vi "例13.2 仿真信号的生成.vi"() -> ()   [LabVIEW 2017]
uses:
  <vilib>/measure/NI_MABase.lvlib
  <vilib>/measure/NI_MAPro.lvlib
panel:
  in  "相位":dbl
  in  "幅值":dbl
  in  "频率":dbl
  in  "停止":bool
  in  "formula":string="sin(w*t)*sin(2*pi(1)*t)" caption="公式"
  in  "噪声选择":enum16{"无", "均匀白噪声", "高斯噪声"}(ring)
  in  "波形选择":enum16{"正弦波", "三角波", "方波", "公式波"}(ring)
  in  "信噪比":dbl=1.0 format="%.2p"
  in  "square wave \nduty cycle (%)":dbl=50.0 caption="方波占空比(%)" format="%0.2f"
  in  "sampling info":cluster{"Fs":dbl, "#s":dbl}={"Fs"=1000.0, "#s"=1000.0} caption="采样信息" {"Fs" format="%.2p"}
  out "波形图":waveform(dbl)(graph)
  # "波 形 发 生 器"
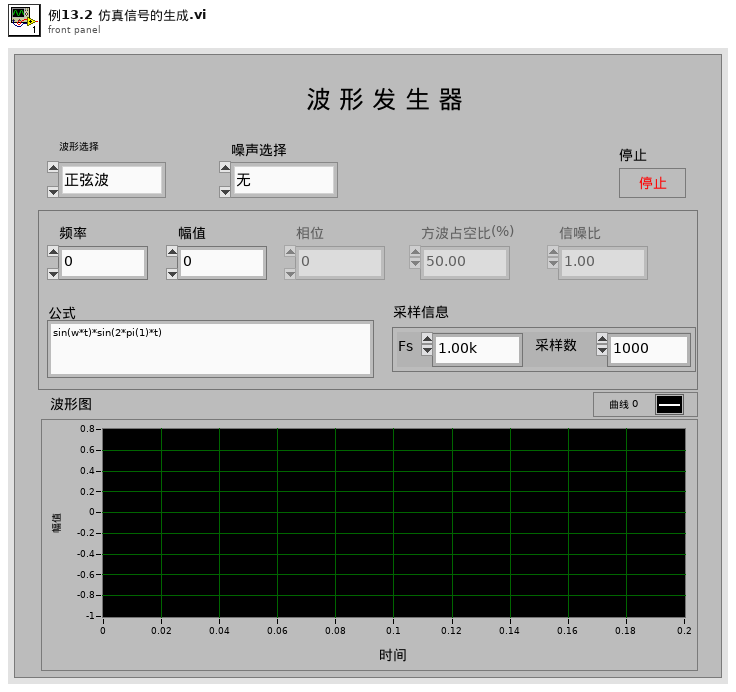
[diagram p1: front panel]
types:
  T1 = enum8{"Enabled", "Disabled", "Disabled and Grayed Out"}
  T2 = enum16{"Sine Wave", "Triangle Wave", "Square Wave", "Sawtooth Wave"}
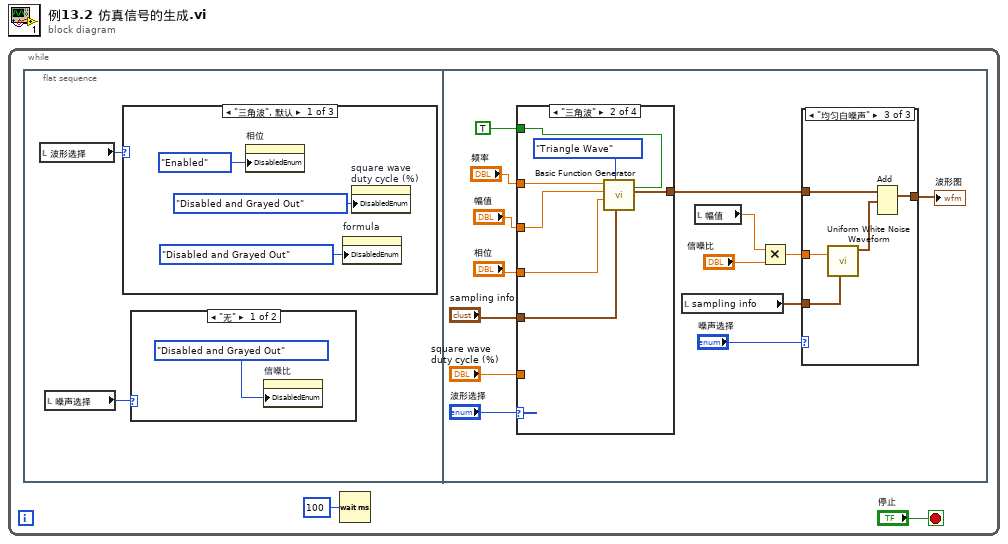
[diagram p0: block diagram]
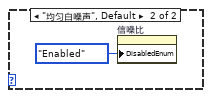
[diagram p2: hidden frame]
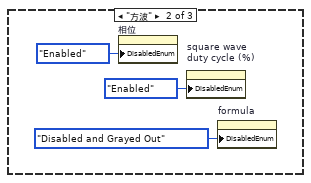
[diagram p3: hidden frame]
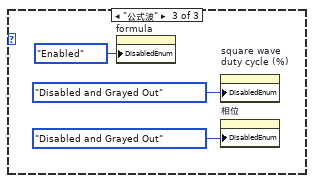
[diagram p4: hidden frame]
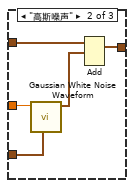
[diagram p6: hidden frame]
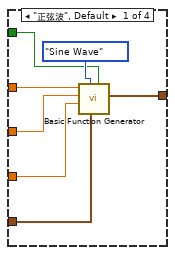
[diagram p7: hidden frame]
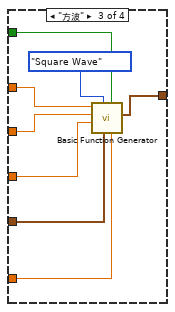
[diagram p8: hidden frame]
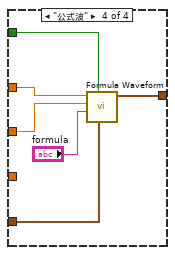
[diagram p9: hidden frame]
diagram:
  n1 = while {
    stop <- "停止" stop-if-true
    n2 = flat-sequence {
      frame #0 {
        n3 = local read "波形选择"() -> (w4:enum16{"正弦波", "三角波", "方波", "公式波"})
        n4 = local read "噪声选择"() -> (w3:enum16{"无", "均匀白噪声", "高斯噪声"})
        n5 = case shown="\"三角波\", 默认" w4 {
          frame "三角波", Default {
            n6 = property on="相位" class="DigNum (严格)"("DisabledEnum"=T1."Enabled" ("禁用")) -> ()  [unwired: 2 in, 2 out]
            n7 = property on="formula" class="Str"("DisabledEnum"=T1."Disabled and Grayed Out" ("禁用")) -> ()  [unwired: 2 in, 2 out]
            n8 = property on="square wave \nduty cycle (%)" class="DigNum (严格)"("DisabledEnum"=T1."Disabled and Grayed Out" ("禁用")) -> ()  [unwired: 2 in, 2 out]
          }
          frame "方波" {
            n9 = property on="相位" class="DigNum (严格)"("DisabledEnum"=T1."Enabled" ("禁用")) -> ()  [unwired: 2 in, 2 out]
            n10 = property on="square wave \nduty cycle (%)" class="DigNum (严格)"("DisabledEnum"=T1."Enabled" ("禁用")) -> ()  [unwired: 2 in, 2 out]
            n11 = property on="formula" class="Str"("DisabledEnum"=T1."Disabled and Grayed Out" ("禁用")) -> ()  [unwired: 2 in, 2 out]
          }
          frame "公式波" {
            n12 = property on="formula" class="Str"("DisabledEnum"=T1."Enabled" ("禁用")) -> ()  [unwired: 2 in, 2 out]
            n13 = property on="square wave \nduty cycle (%)" class="DigNum (严格)"("DisabledEnum"=T1."Disabled and Grayed Out" ("禁用")) -> ()  [unwired: 2 in, 2 out]
            n14 = property on="相位" class="DigNum (严格)"("DisabledEnum"=T1."Disabled and Grayed Out" ("禁用")) -> ()  [unwired: 2 in, 2 out]
          }
        }
        n15 = case shown="\"无\"" w3 {
          frame "无" {
            n16 = property on="信噪比" class="DigNum (严格)"("DisabledEnum"=T1."Disabled and Grayed Out" ("禁用")) -> ()  [unwired: 2 in, 2 out]
          }
          frame "均匀白噪声", Default {
            n17 = property on="信噪比" class="DigNum (严格)"("DisabledEnum"=T1."Enabled" ("禁用")) -> ()  [unwired: 2 in, 2 out]
          }
        }
      }
      frame #1 {
        n18 = case shown="\"三角波\"" "波形选择" {
          tunnel: [w43 w54 w56 w65] -> w27
          tunnel: "频率" -> [w46 w52 w61 w68]
          tunnel: "幅值" -> [w45 w51 w60 w67]
          tunnel: "相位" -> [w42 w50 w59 _]
          tunnel: "sampling info" -> [w44 w49 w58 w64]
          tunnel: "square wave \nduty cycle (%)" -> [_ _ w57 _]
          tunnel: TRUE ("reset signal") -> [w41 w48 w55 w63]
          frame "正弦波", Default {
            n19 = call <vilib>:"Basic Function Generator.vi"("reset signal"=w41, "sampling info"=w44, "signal type"=T2."Sine Wave", "phase"=w42, "amplitude"=w45, "frequency"=w46) -> ("signal out"=w43:waveform(dbl))  [unwired: 3 in, 2 out]
          }
          frame "三角波" {
            n20 = call <vilib>:"Basic Function Generator.vi"("reset signal"=w48, "sampling info"=w49, "signal type"=T2."Triangle Wave", "phase"=w50, "amplitude"=w51, "frequency"=w52) -> ("signal out"=w54:waveform(dbl))  [unwired: 3 in, 2 out]
          }
          frame "方波" {
            n21 = call <vilib>:"Basic Function Generator.vi"("square wave duty cycle (%)"=w57, "reset signal"=w55, "sampling info"=w58, "signal type"=T2."Square Wave", "phase"=w59, "amplitude"=w60, "frequency"=w61) -> ("signal out"=w56:waveform(dbl))  [unwired: 2 in, 2 out]
          }
          frame "公式波" {
            n22 = call <vilib>:"Formula Waveform.vi"("sampling info"=w64, "reset signal"=w63, "formula"="formula", "amplitude"=w67, "frequency"=w68) -> ("signal out"=w65:waveform(dbl))  [unwired: 5 in, 1 out]
          }
        }
        n23 = local read "sampling info"() -> (w19:cluster{"Fs":dbl, "#s":dbl})
        n24 = local read "幅值"() -> (w28:dbl)
        n25 = Multiply(x=w28, y="信噪比") -> (x*y=w26:dbl)
        n26 = case shown="\"均匀白噪声\"" "噪声选择" {
          tunnel: [w30 w34 w37] -> w16
          tunnel: w26 -> [_ w35 w40]
          tunnel: w27 -> [w30 w33 w39]
          tunnel: w19 -> [_ w32 w36]
          frame "无", Default {
          }
          frame "高斯噪声" {
            n27 = call <vilib>:"Gaussian White Noise Waveform.vi"("sampling info"=w32, "standard deviation"=w35) -> ("signal out"=w31:waveform(dbl))  [unwired: 8 in, 1 out]
            n28 = Add(1:w31, 2:w33) -> (0:w34:waveform(dbl))  [unwired: 1 in, 1 out]
          }
          frame "均匀白噪声" {
            n29 = call <vilib>:"Uniform White Noise Waveform.vi"("sampling info"=w36, "amplitude"=w40) -> ("signal out"=w38:waveform(dbl))  [unwired: 8 in, 1 out]
            n30 = Add(1:w38, 2:w39) -> (0:w37:waveform(dbl))  [unwired: 1 in, 1 out]
          }
        }
        "波形图" <- w16
      }
    }
    n31 = Wait (ms)(milliseconds to wait=u32 100 ("等待时间（毫秒）")) -> ()  [unwired: 1 out]
  }
